vi "Get camera handle.vi"(8 "error in (no error)":errorcluster, 11 "DAQMH121119OrcaFlash in":refnum<class "DAQOrcaFlash.lvclass">) -> (0 "error out":errorcluster, 2 "cam handle":u32, 3 "DAQMH121119OrcaFlash out":refnum<class "DAQOrcaFlash.lvclass">)   [LabVIEW 2012, in "DAQOrcaFlash.lvclass"]
uses:
  DAQOrcaFlash.lvclass
  DAQOrcaFlash.lvclass/DAQOrcaFlash.ctl
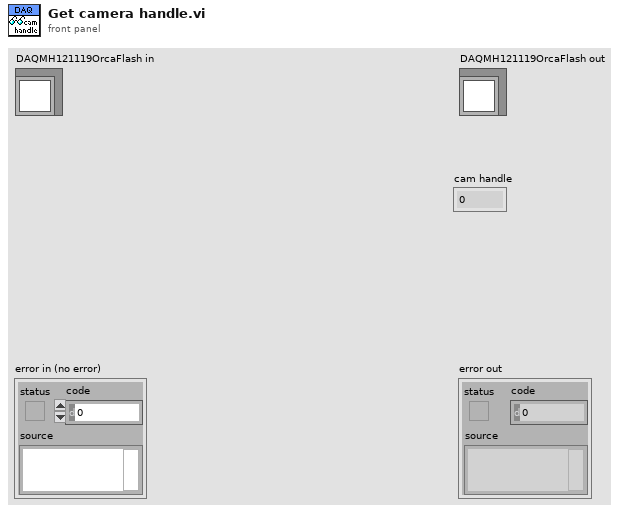
[diagram p1: front panel]
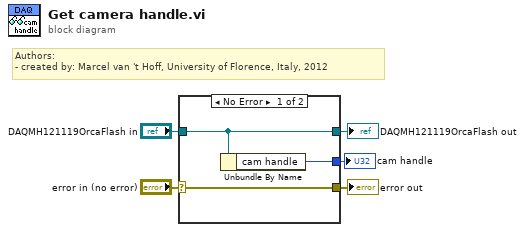
[diagram p0: block diagram]
diagram:
  # "Authors: \n- created by: Marcel van 't Hoff, University of Florence, Italy, 2012"
  n1 = case shown="No Error" "error in (no error)" {
    selector: "error in (no error)" -> [w8 w10]
    tunnel: [w8 w10] -> w4
    tunnel: [w7 w9] -> w2
    tunnel: "DAQMH121119OrcaFlash in" -> [w7 w9]
    tunnel: [w6 _] -> w1
    frame No Error {
      n2 = Unbundle By Name(w7) -> ("cam handle"=w6:u32)
    }
    frame Error {
    }
  }
  "error out" <- w4
  "DAQMH121119OrcaFlash out" <- w2
  "cam handle" <- w1
